vi "Wait For Bytes.vi"(0 "VISA resource":refnum<visa-resource-name>, 5 "Bytes To Read":u32, 9 "Time Out (100 ms)":i32=100, 11 "error in":errorcluster) -> (4 "VISA resource":refnum<visa-resource-name>, 8 "Bytes Available?":bool, 15 "error out":errorcluster)   [LabVIEW 2011, in "LabVIEW Interface for Arduino.lvlib"]
doc: "Wait for the specified number of bytes to be available in the VISA buffer."
uses:
  <vilib>/LabVIEW Interface for Arduino/LabVIEW Interface for Arduino.lvlib
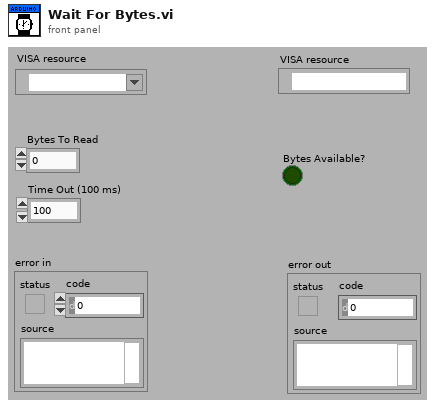
[diagram p1: front panel]
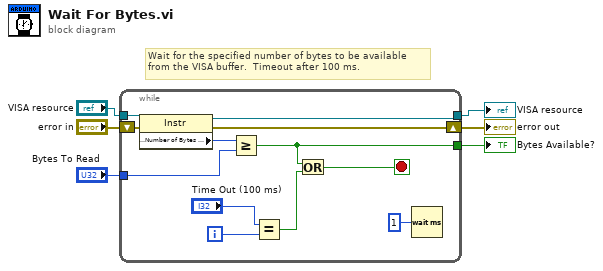
[diagram p0: block diagram]
diagram:
  # "Wait for the specified number of bytes to be available\nfrom the VISA buffer.  Timeout after 100 ms."
  n1 = while {
    tunnel: "Bytes To Read" -> [w11]
    tunnel: [w18] -> w4
    tunnel: "VISA resource" -> [w14]
    shift-right: [w10] -> w2
    shift-left: "error in" -> [w13]
    tunnel: [w7] -> w1
    i -> [w16]
    stop <- w8 stop-if-true
    n2 = property class="Instr"(reference=w14, error in=w13) -> (reference out=w18:refnum<visa-resource-name>, error out=w10:errorcluster, "Serial Settings:Number of Bytes at Serial Port"=w12:u32)
    n3 = Greater Or Equal?(x=w12, y=w11) -> (x >= y?=w7:bool)
    n4 = Equal?(x="Time Out (100 ms)", y=w16) -> (x = y?=w9:bool)
    n5 = Or(x=w7, y=w9) -> (x .or. y?=w8:bool)
    n6 = Wait (ms)(milliseconds to wait=u32 1) -> ()  [unwired: 1 out]
  }
  "VISA resource" <- w4
  "error out" <- w2
  "Bytes Available?" <- w1
